vi "DMA WriteMod3.vi"(8 "error in (no error)":errorcluster, 10 "number of elements":u32, 11 "Refnum in":refnum<k20>) -> (0 "error out":errorcluster, 1 "peak fullness":u32, 2 "fullness":u32, 3 "Refnum out":refnum<k20>, 4 "empty elements remaining":u32, 5 "Write Region Reference":refnum<data-value>)   [LabVIEW 2017]
uses:
  <vilib>/Utility/error.llb/Error Cluster From Error Code.vi
  <vilib>/rvi/errors/niLvFpgaAdjustHostInterfaceError.vi
  <vilib>/rvi/interface/nirviMethod/nirviMethod.xnode
  <vilib>/rvi/interface/nirviReadWriteControl/nirviReadWriteControl.xnode
  NiFpgaLv.dll
  <vilib>/rvi/interface/Simulation/niFpgaSimulationCallBeginRW.vi
  <vilib>/rvi/errors/niLvFpgaMergeErrorWithErrorCode.vi
  <vilib>/FPGAPlugInAG/Dynamic/niLvFpga_AcquireWriteRegionFifo_Dynamic.vi
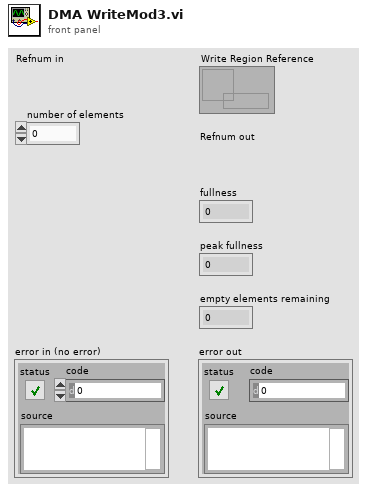
[diagram p1: front panel]
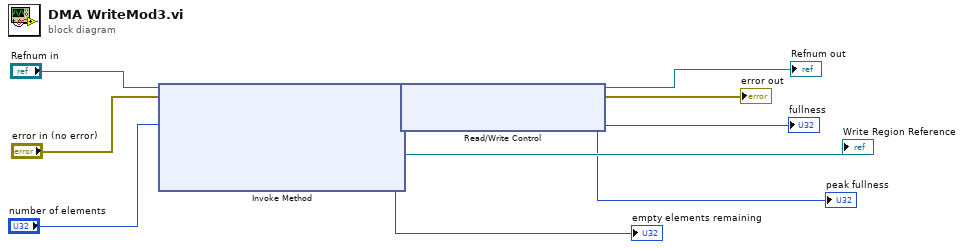
[diagram p0: block diagram]
diagram:
  n1 = xnode "Invoke Method"("FPGA VI Reference In"="Refnum in", "error in"="error in (no error)", "Number of Elements"="number of elements") -> ("FPGA VI Reference Out"=w9:refnum<k20>, "error out"=w10:errorcluster, "Write Region Reference"=→"Write Region Reference":refnum<data-value>, "Empty Elements Remaining"=→"empty elements remaining":u32)  [unwired: 1 in, 1 out]
  n2 = xnode "Read/Write Control"("FPGA VI Reference In"=w9, "error in"=w10) -> ("FPGA VI Reference Out"=→"Refnum out":refnum<k20>, "error out"=→"error out":errorcluster, "streaming output.dma fullness"=→"fullness":u32, "streaming output.dma min elements"=→"peak fullness":u32)
